vi "数据库插入_B030.vi"(0 "壳体条码":string="PPPPPP") -> ()   [LabVIEW 2013]
panel:
  out "error out":errorcluster
  out "eof":bool
  in  "error in (no error) 2":errorcluster
  # "1-10"
  # "1-6"
  # "1-40"
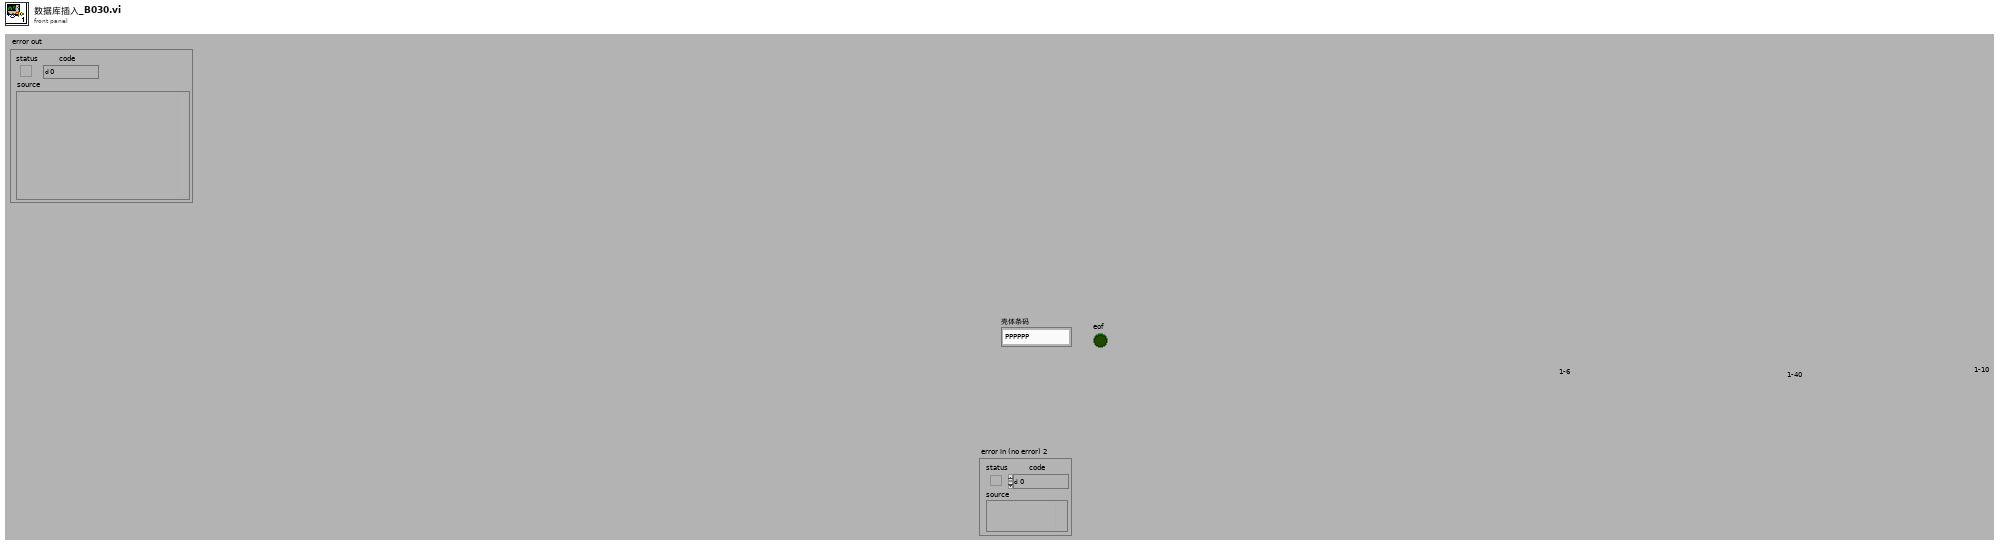
[diagram p1: front panel]
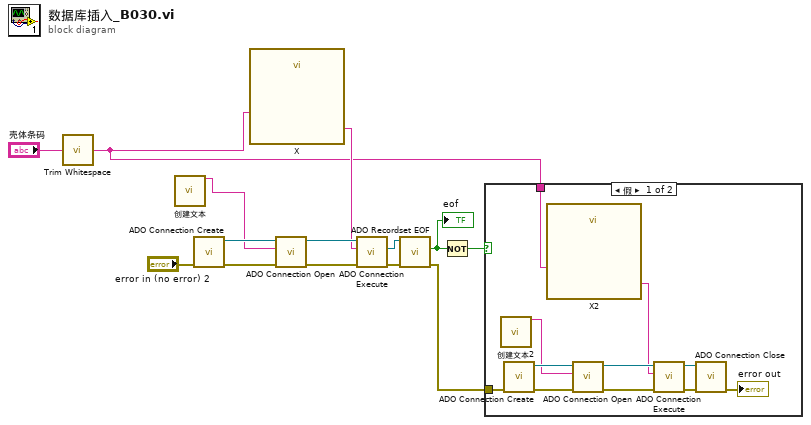
[diagram p0: block diagram]
diagram:
  n1 = call <vilib>:"Trim Whitespace.vi"("string"="壳体条码") -> ("trimmed string"=w3:string)  [unwired: 1 in]
  n2 = call "创建文本"() -> ("Result"=w2:string)  [unwired: 14 in, 1 out]
  n3 = call "ADO Connection Create.vi"("error in (no error)"="error in (no error) 2") -> ("error out"=w13:errorcluster, "ADODB._Connection Out"=w12:refnum<k7>)  [unwired: 9 out]
  n4 = call "X"("壳体条码"=w3) -> ("Result"=w9:string)  [unwired: 13 in, 1 out]
  n5 = call "ADO Connection Open.vi"("error in (no error)"=w13, "ConnectionString"=w2, "ADODB._Connection In"=w12) -> ("error out"=w11:errorcluster, "ADODB._Connection Out"=w10:refnum<k7>)  [unwired: 7 out]
  n6 = call "ADO Connection Execute.vi"("error in (no error)"=w11, "CommandText"=w9, "ADODB._Connection In"=w10) -> ("error out"=w7:errorcluster, "RecordSet"=w8:refnum<k7>)  [unwired: 7 out]
  n7 = call "ADO Recordset EOF.vi"("error in (no error)"=w7, "ADODB._Recordset In"=w8) -> ("error out"=w1:errorcluster, "EOF"=w6:bool)  [unwired: 7 in, 1 out]
  "eof" <- w6
  n8 = Not(x=w6) -> (.not. x?=w5:bool)
  n9 = case shown="假" w5 {
    tunnel: w3 -> [w17 _]
    tunnel: w1 -> [w15 _]
    frame False {
      n10 = call "创建文本2"() -> ("Result"=w16:string)  [unwired: 14 in, 1 out]
      n11 = call "ADO Connection Create.vi"("error in (no error)"=w15) -> ("error out"=w22:errorcluster, "ADODB._Connection Out"=w21:refnum<k7>)  [unwired: 9 out]
      n12 = call "X2"("壳体条码"=w17) -> ("Result"=w18:string)  [unwired: 13 in, 1 out]
      n13 = call "ADO Connection Open.vi"("error in (no error)"=w22, "ConnectionString"=w16, "ADODB._Connection In"=w21) -> ("error out"=w20:errorcluster, "ADODB._Connection Out"=w19:refnum<k7>)  [unwired: 7 out]
      n14 = call "ADO Connection Execute.vi"("error in (no error)"=w20, "CommandText"=w18, "ADODB._Connection In"=w19) -> ("error out"=w24:errorcluster, "ADODB._Connection Out"=w23:refnum<k7>)  [unwired: 7 out]
      n15 = call "ADO Connection Close.vi"("error in (no error)"=w24, "ADODB._Connection In"=w23) -> ("error out"=→"error out":errorcluster)  [unwired: 9 out]
    }
    frame True {
    }
  }
